vi "Create Message - Value Change & Trigger.vi"(7 "optional settings":T2={"Protection"=enum."None", "Enable Periodic Default"=FALSE, "Trigger Channel refnum"=18446744073709551615} {"Trigger Channel refnum" format="%x"}, 8 "error in (no error)":errorcluster, 10 "message name":string, 11 "message group refnum in":T1=18446744073709551615 format="%.0x") -> (0 "error out":errorcluster, 2 "message refnum out":T1 format="%.0x", 3 "message group refnum out":T1 format="%.0x")   [LabVIEW 2020, in "Instrument Addon Scripting API.lvlib"]
doc: "Creates a new message section that sets the Generation Type to Value Change & Trigger. \n\nValue Change & Trigger will cause the message to appear based on the Trigger Channel or anytime a command field channel changes value. If the command message contains multiple VeriStand channels, the message will be sent each time one of the channels has changes."
uses:
  Instrument Addon Scripting API.lvlib
  TypeDefs/Message Settings.ctl
  TypeDefs/Protection Types.ctl
  <vilib>/NI VeriStand/Custom Device API/Custom Device Item Ref.ctl
  <vilib>/NI VeriStand/Custom Device API/Custom Device Channel.ctl
  <vilib>/NI VeriStand/Custom Device API/Custom Device Channel Type.ctl
  Shared Directory/Message Generation Type.ctl
  <vilib>/NI VeriStand/Custom Device API/Custom Device API.lvlib
  Shared Directory/Instrument Addon Shared.lvlib
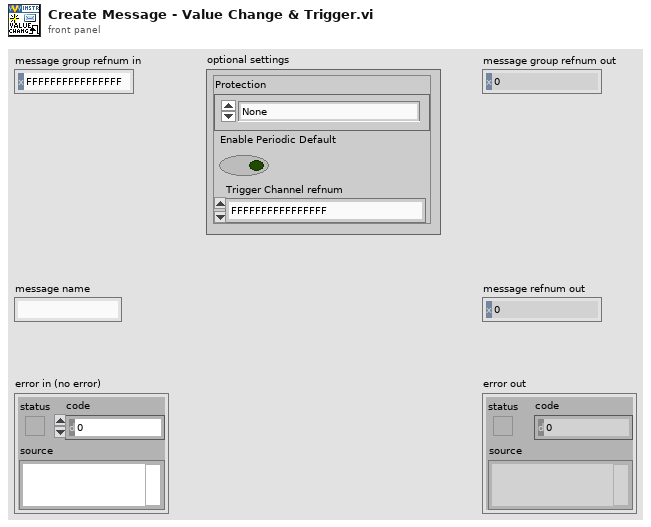
[diagram p1: front panel]
types:
  T1 = typedef "Custom Device API.lvlib/Custom Device Item Ref.ctl" = u64
  T2 = typedef "Instrument Addon Scripting API.lvlib/Message Settings.ctl" = cluster{"Protection":T3, "Enable Periodic Default":bool, "Trigger Channel refnum":u64}
  T3 = typedef "Instrument Addon Scripting API.lvlib/Protection Types.ctl" = enum16{"None", "CRC-32", "Checksum U16", "Checksum U32", "Checksum U8"}
  T4 = typedef "Instrument Addon Shared.lvlib/Message Generation Type.ctl" = enum16{"Trigger Only", "Periodic & Trigger", "Value Change & Trigger"}
  T5 = typedef "Custom Device API.lvlib/Custom Device Channel.ctl" = cluster{"Type":T6, "Units":string, "Default Value":dbl, "Faultable":bool, "Scalable":bool}
  T6 = typedef "Custom Device API.lvlib/Custom Device Channel Type.ctl" = enum16{"Input", "Output"}
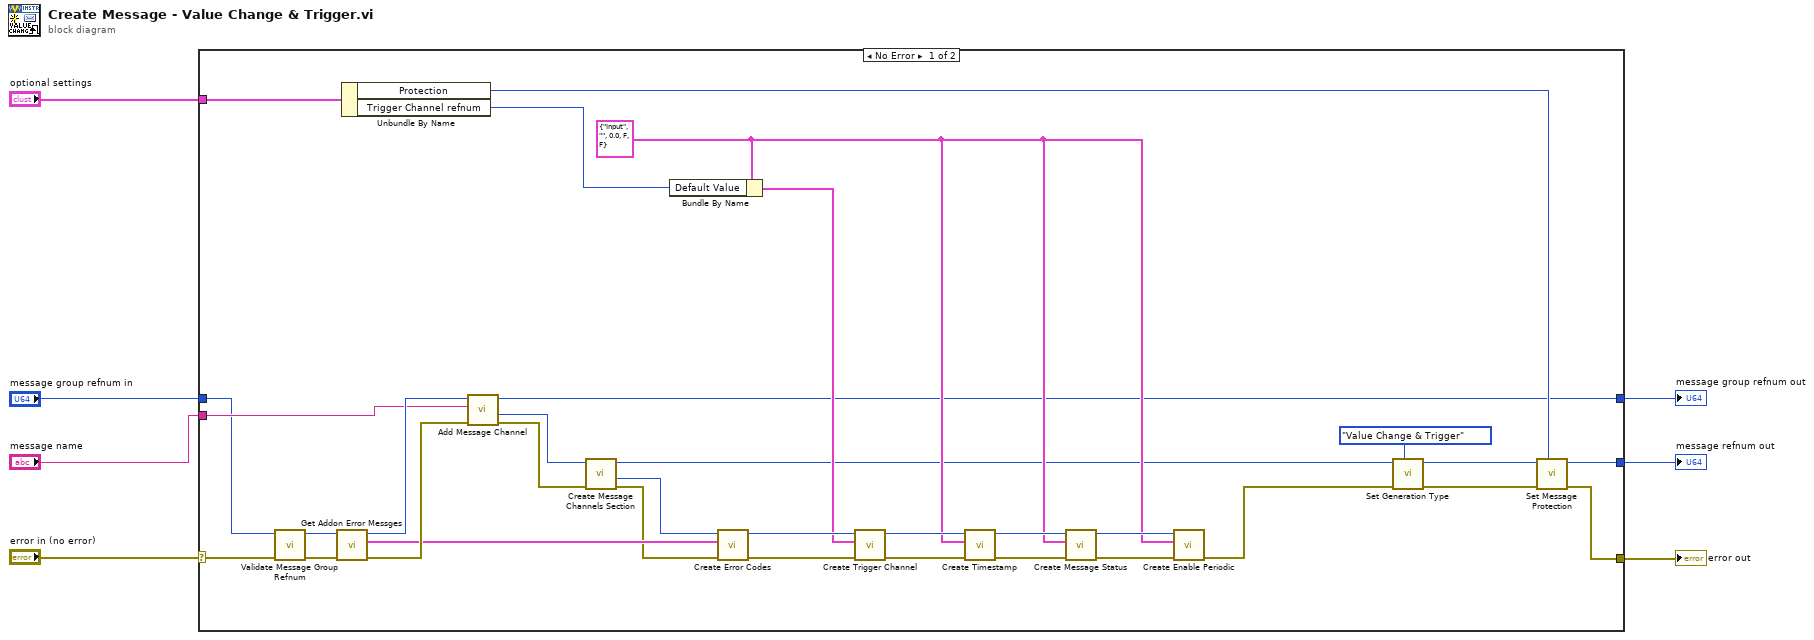
[diagram p0: block diagram]
diagram:
  n1 = case shown="No Error" "error in (no error)" {
    selector: "error in (no error)" -> [w10 w42]
    tunnel: [w21 w42] -> w7
    tunnel: "optional settings" -> [w17 _]
    tunnel: "message name" -> [w16 _]
    tunnel: [w15 w41] -> w4
    tunnel: [w14 _] -> w3
    tunnel: "message group refnum in" -> [w9 w41]
    frame No Error {
      w20 = T5 {"Type"=enum."Input", "Units"="", "Default Value"=0.0, "Faultable"=FALSE, "Scalable"=FALSE} ("Channel")
      n2 = call "Validate Message Group Refnum.vi"("error in (no error)"=w10, "message group refnum in"=w9) -> ("error out"=w11:errorcluster, "message group refnum out"=w8:T1)  [unwired: 8 in]
      n3 = call "Get Addon Error Messges.vi"("error in (no error)"=w11, "Message Group in"=w8) -> ("error out"=w36:errorcluster, "Error Messages out"=w33:cluster{"Code":i32, "String":string}[], "Message Group out"=w32:u64)  [unwired: 7 in]
      n4 = Unbundle By Name(w17) -> ("Protection"=w22:T3, "Trigger Channel refnum"=w18:u64)
      n5 = call "Add Message Channel.vi"("error in (no error)"=w36, "Message Name"=w16, "Message Group in"=w32) -> ("error out"=w40:errorcluster, "Message out"=w34:T1, "Message Group out"=w15:T1)  [unwired: 6 in]
      n6 = call "Create Message Channels Section.vi"("error in (no error)"=w40, "Message in"=w34) -> ("error out"=w31:errorcluster, "Message Channels Section out"=w30:T1, "Message out"=w12:T1)  [unwired: 7 in]
      n7 = Bundle By Name(cluster=w20, "Default Value"=w18) -> (w19:T5)
      n8 = call "Create Error Codes.vi"("error in (no error)"=w31, "Error Codes"=w33, "Message Channels Section in"=w30) -> ("error out"=w28:errorcluster, "Message Channels Section out"=w29:T1)  [unwired: 7 in]
      n9 = call "Create Trigger Channel.vi"("error in (no error)"=w28, "Channel Parameters"=w19, "Message Channels Section in"=w29) -> ("error out"=w27:errorcluster, "Message Channels Section out"=w26:T1)  [unwired: 6 in, 1 out]
      n10 = call "Create Timestamp.vi"("error in (no error)"=w27, "Channel Paramters"=w20, "Message Channels Section in"=w26) -> ("error out"=w39:errorcluster, "Message Channels Section out"=w35:T1)  [unwired: 6 in, 1 out]
      n11 = call "Create Message Status.vi"("error in (no error)"=w39, "Channel Paramters"=w20, "Message Channels Section in"=w35) -> ("error out"=w38:errorcluster, "Message Channels Section out"=w37:T1)  [unwired: 7 in]
      n12 = call "Create Enable Periodic.vi"("error in (no error)"=w38, "Channel Parameters"=w20, "Message Channels Section in"=w37) -> ("error out"=w13:errorcluster)  [unwired: 7 in, 1 out]
      n13 = call "Set Generation Type.vi"("Generation Type"=Message_Generation_Type."Value Change & Trigger", "error in (no error)"=w13, "Message in"=w12) -> ("error out"=w24:errorcluster, "Message out"=w23:T1)  [unwired: 7 in]
      n14 = call "Set Message Protection.vi"("Protection Type"=w22, "error in (no error)"=w24, "Message in"=w23) -> ("error out"=w21:errorcluster, "Message out"=w14:T1)  [unwired: 7 in]
    }
    frame Error {
    }
  }
  "error out" <- w7
  "message group refnum out" <- w4
  "message refnum out" <- w3
